vi "读取NPLC.vi"(8 "error in (no error)":errorcluster caption="错误输入（无错误）", 11 "Keithley 2000输入":refnum<class "Keithley 2000.lvclass">) -> (0 "error out":errorcluster caption="错误输出", 2 "NPLC":dbl=1.0, 3 "Keithley 2000输出":refnum<class "Keithley 2000.lvclass">)   [LabVIEW 2020, in "DMM.lvlib" / "Keithley 2000.lvclass"]
uses:
  Keithley 2000.lvclass
  Keithley 2000.lvclass/Keithley 2000.ctl
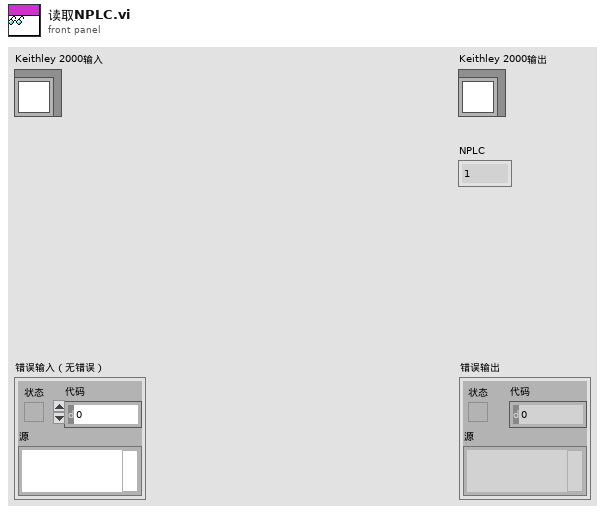
[diagram p1: front panel]
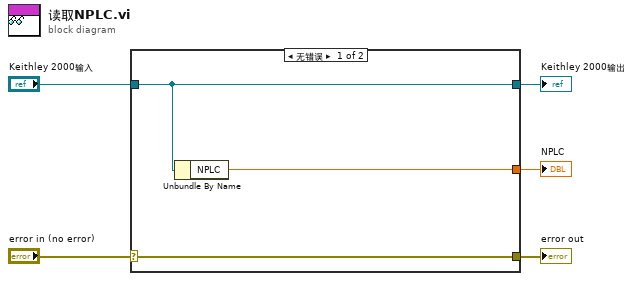
[diagram p0: block diagram]
diagram:
  n1 = case shown="无错误" "error in (no error)" {
    selector: "error in (no error)" -> [w8 w9]
    tunnel: [w8 w9] -> w4
    tunnel: [w7 w10] -> w2
    tunnel: "Keithley 2000输入" -> [w7 w10]
    tunnel: [w6 _] -> w1
    frame No Error {
      n2 = Unbundle By Name(w7) -> ("NPLC"=w6:dbl)
    }
    frame Error {
    }
  }
  "error out" <- w4
  "Keithley 2000输出" <- w2
  "NPLC" <- w1
